vi "RS232ComPort Init.vi"(8 "error in (no error)":errorcluster) -> (0 "error out":errorcluster, 3 "RS232ComPort out":refnum<class "RS232ComPort.lvclass">)   [LabVIEW 2018, in "RS232ComPort.lvclass"]
uses:
  RS232ComPort.lvclass
  RS232ComPort.lvclass/RS232ComPort.ctl
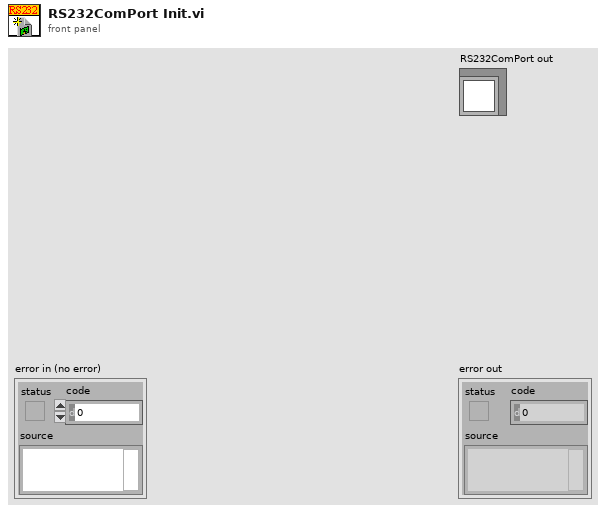
[diagram p1: front panel]
types:
  T1 = typedef "Semaphore RefNum" = refnum<k1>
  T2 = cluster{"Response Str":string, "VISA resource":refnum<visa-resource-name>, "DeviceExist?":bool, "semaphore":T1}
  T3 = cluster{"Response Str":string, "VISA resource":refnum<visa-resource-name>, "DeviceExist?":bool, "semaphore":T1}[]
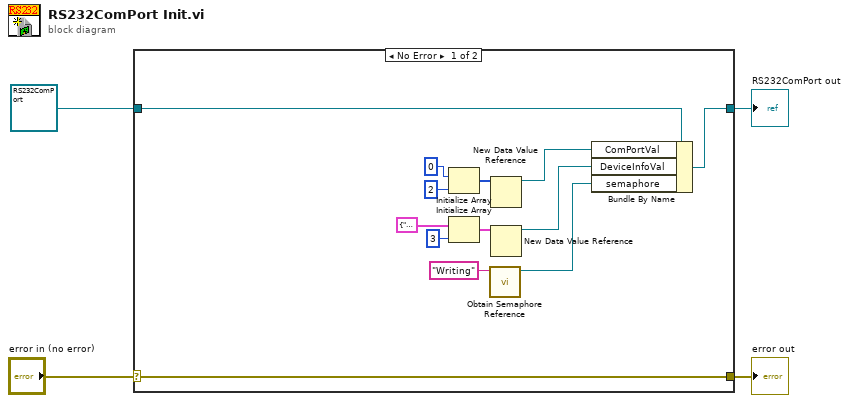
[diagram p0: block diagram]
diagram:
  n1 = case shown="No Error" "error in (no error)" {
    selector: "error in (no error)" -> [w16 w19]
    tunnel: [w16 w19] -> w3
    tunnel: [w11 w18] -> w1
    tunnel: refnum<class "RS232ComPort.lvclass"> refnum ("RS232ComPort in") -> [w17 w18]
    frame No Error {
      n2 = Initialize Array(i8 0, 2 ("dimension size")) -> (w9:i8[])
      n3 = Initialize Array(T2 {"Response Str"="", "VISA resource"="", "DeviceExist?"=FALSE, "semaphore"=refnum}, 3 ("dimension size")) -> (w10:T3)
      n4 = call <vilib>:"Obtain Semaphore Reference.vi"("name (unnamed)"="Writing") -> ("semaphore"=w5:T1)  [unwired: 4 in, 2 out]
      n5 = New Data Value Reference(data value=w9) -> (data value reference=w8:refnum<data-value>)  [unwired: 1 in, 1 out]
      n6 = New Data Value Reference(data value=w10) -> (data value reference=w7:refnum<data-value>)  [unwired: 1 in, 1 out]
      n7 = Bundle By Name(cluster=w17, "ComPortVal"=w8, "DeviceInfoVal"=w7, "semaphore"=w5) -> (w11:refnum<class "RS232ComPort.lvclass">)
    }
    frame Error {
    }
  }
  "error out" <- w3
  "RS232ComPort out" <- w1
